vi "Multicast Receiver & RIO Sender AllKF.vi"() -> (1 "Fusion Data":dbl, 3 "Multicast":dbl[][](graph))   [LabVIEW 2015]
doc: "Creates a read-only UDP multicast session and receives data on the specified port."
uses:
  <vilib>/Utility/tcp.llb/UDP Multicast Read-Only Open.vi
panel:
  out "Local KFs and Fusion KF":dbl[][](graph)
  out "KF_Kinect2":dbl
  out "KF_Xbox Data":dbl
  out "error out":errorcluster
  in  "Stop":bool
  # "Overview: Demonstrates the use of the UDP functions to connect to a UDP multicast session and receive data.\nInstructions:\n1. Ensure UDP Multicast - Sender.vi is already running.\n2. Run the VI.\n3. Click Stop to stop the VI."
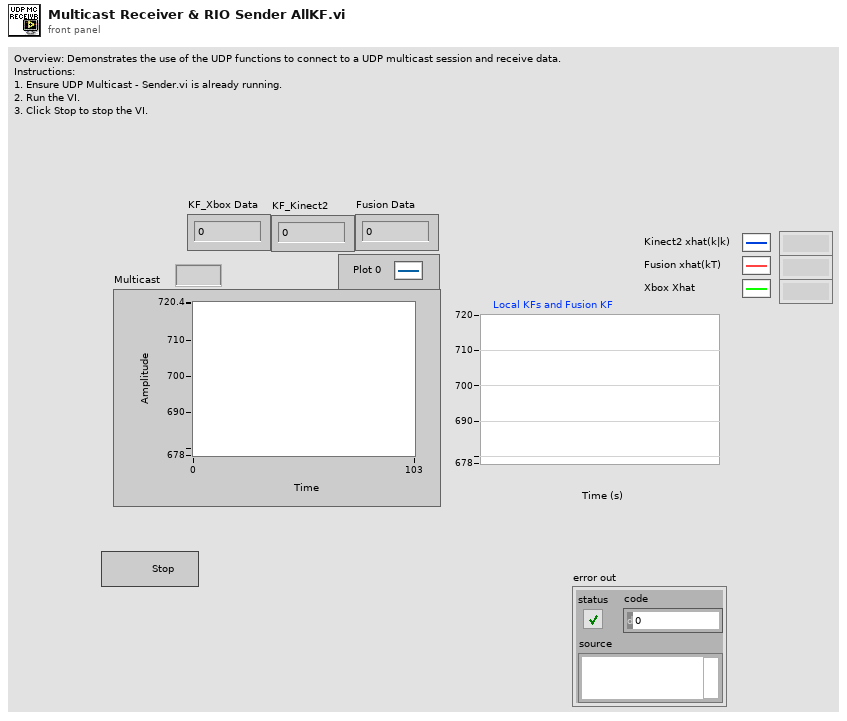
[diagram p1: front panel]
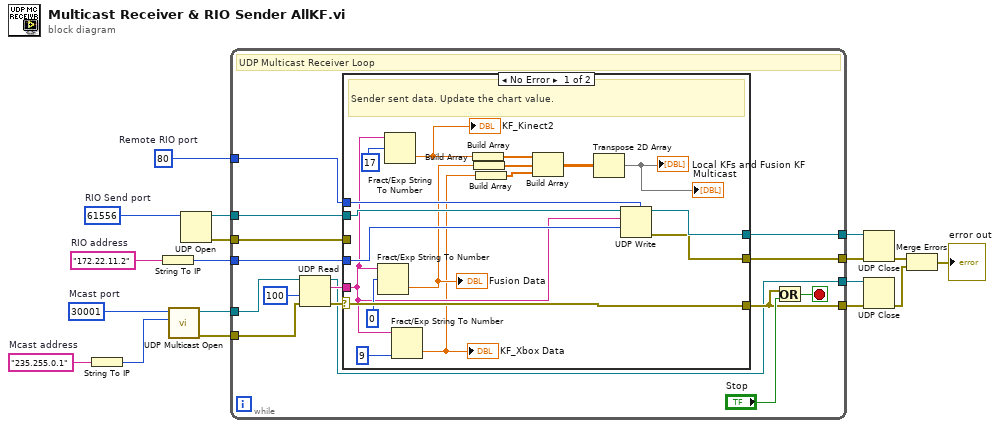
[diagram p0: block diagram]
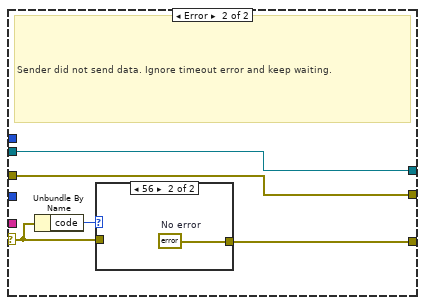
[diagram p2: hidden frame]
diagram:
  w6 = u16 80  # Remote RIO port
  w10 = u16 61556  # RIO Send port
  w11 = "172.22.11.2"  # RIO address
  w13 = u16 30001  # Mcast port
  w17 = "235.255.0.1"  # Mcast address
  n1 = String To IP(1:w17) -> (0:w12:u32)
  n2 = String To IP(1:w11) -> (0:w7:u32)
  n3 = call-poly <vilib>:"UDP Multicast Open.vi"("multicast addr"=w12, "port"=w13) -> ("error out"=w15:errorcluster, "connection ID"=w14:refnum<k16>)  [unwired: 7 in, 1 out]
  n4 = UDP Open(11:w10) -> (port=w8:refnum<k16>, 0:w9:errorcluster)  [unwired: 4 in, 1 out]
  n5 = while {
    tunnel: w14 -> [w33]
    tunnel: [w25] -> w18
    tunnel: w15 -> [w30]
    tunnel: [w26] -> w16
    tunnel: w9 -> [w19]
    tunnel: w8 -> [w24]
    tunnel: w7 -> [w23]
    tunnel: w6 -> [w22]
    tunnel: [w21] -> w5
    tunnel: [w20] -> w4
    stop <- w31 stop-if-true
    # "UDP Multicast Receiver Loop"
    n6 = UDP Read(connection ID=w33, timeout ms (25000)=100, 8:w30) -> (data out=w28:string, error out=w27:errorcluster, 3:w25:refnum<k16>)  [unwired: 3 out]
    n7 = case shown="No Error" w27 {
      selector: w27 -> [w46 w55]
      tunnel: w28 -> [w42 _]
      tunnel: [w46 w54] -> w26
      tunnel: w24 -> [w51 w53]
      tunnel: w23 -> [w50 _]
      tunnel: w22 -> [w49 _]
      tunnel: [w48 w53] -> w21
      tunnel: [w47 w52] -> w20
      tunnel: w19 -> [_ w52]
      frame No Error {
        # "Sender sent data. Update the chart value."
        n8 = Fract/Exp String To Number(string=w42, offset=0) -> (number=w39:dbl)  [unwired: 2 in, 1 out]
        "Fusion Data" <- w39
        n9 = Fract/Exp String To Number(string=w42, offset=17) -> (number=w41:dbl)  [unwired: 2 in, 1 out]
        "KF_Kinect2" <- w41
        n10 = Fract/Exp String To Number(string=w42, offset=9) -> (number=w37:dbl)  [unwired: 2 in, 1 out]
        "KF_Xbox Data" <- w37
        n11 = Build Array(w41) -> (w40:dbl[])
        n12 = Build Array(w39) -> (w38:dbl[])
        n13 = Build Array(w37) -> (w36:dbl[])
        n14 = Build Array(w40, w38, w36) -> (w35:dbl[][])
        n15 = Transpose 2D Array(2D array=w35) -> (transposed array=→"Local KFs and Fusion KF" →"Multicast":dbl[][])
        n16 = UDP Write(address=w50, port or service name=w49, connection ID=w51, data in=w42) -> (error out=w47:errorcluster, 3:w48:refnum<k16>)  [unwired: 2 in]
      }
      frame Error {
        # "Sender did not send data. Ignore timeout error and keep waiting."
        n17 = Unbundle By Name(w55) -> ("code"=w56:i32)
        n18 = case shown="56" w56 {
          tunnel: w55 -> [w57 _]
          tunnel: [w57 w58] -> w54
          frame Default {
          }
          frame 56 {
            w58 = errorcluster {"status"=FALSE, "code"=0, "source"=""}  # No error
          }
        }
      }
    }
    n19 = Or(x=w26, y="Stop") -> (x .or. y?=w31:bool)
  }
  n20 = UDP Close(connection ID=w5, 8:w4) -> (error out=w3:errorcluster)  [unwired: 1 out]
  n21 = UDP Close(connection ID=w18, 8:w16) -> (error out=w2:errorcluster)  [unwired: 1 out]
  n22 = Merge Errors(w3, w2) -> (→"error out":errorcluster)
